vi "String-Cluster.vi"() -> ()   [LabVIEW 2012]
panel:
  out "Output":i32[](array[numeric])
  out "Input":i64[](array[numeric])
  out "Correlator Initial Data 2":T1={"[0]"=1, "Channel1 Threshold Voltage (mV)"=1, "Channel1 Pulse Front"="", "Channel2 Threshold Voltage (mV)"=1, "Channel2 Pulse Front"="", "Channel3 Threshold Voltage (mV)"=1, "Channel3 Pulse Front "="", "Channel4 Threshold Voltage (mV)"=1, "Channel4 Pulse Front "="", "Single Count Enable"={"Channel1"=FALSE, "Channel2"=FALSE, "Channel3"=FALSE, "Channel4"=FALSE}, "Single Count Max"=1, "Sum Count Enable"={"Channel1"=FALSE, "Channel2"=FALSE, "Channel3"=FALSE, "Channel4"=FALSE}, "Sum Count Max"=1, "Start-Stop1 Multyplex"={"Start Channel"="", "Stop Channel"=""}, "Stop Delay 1 (ns)"=1, "Window Length 1 (ns)"=4, "Window Offset 1 (ns) "=4, "Conditional Correlation 1"="", "Histogram Bin 1"="", "Histogram Start 1 (ns) "=4, "Start-Stop2 Multyplex "={"Start Channel"="", "Stop Channel"=""}, "Stop Delay 2 (ns)"=1, "Window Length 2 (ns) "=4, "Window Offset 2 (ns) "=4, "Conditional Correlation 2"="", "Histogram Bin 2"="", "Histogram Start 2 (ns)  "=4, "Start-Stop3 Multyplex"={"Start Channel"="", "Stop Channel"=""}, "Stop Delay 3 (ns)"=1, "Window Length 3 (ns) "=4, "Window Offset 3 (ns) "=4, "Conditional Correlation 3"="", "Histogram Bin 3"="", "Histogram Start 3 (ns) "=4, "Start-Stop4 Multyplex"={"Start Channel"="", "Stop Channel"=""}, "Stop Delay 4 (ns)"=1, "Window Length 4 (ns)  "=4, "Window Offset 4 (ns) "=4, "Conditional Correlation 4"="", "Histogram Bin 4"="", "Histogram Start 4 (ns)  "=4, "Coincidence Count Enable"={"Start-Stop1"=FALSE, "Start-Stop2"=FALSE, "Start-Stop3"=FALSE, "Start-Stop4"=FALSE}, "Coincidence Count Max"=1, "Coincidence Sum Enable 2"={"Start-Stop1"=FALSE, "Start-Stop2"=FALSE, "Start-Stop3"=FALSE, "Start-Stop4"=FALSE}, "Coincidence Sum Max"=1, "Output Channel Enable"={"Channel1"=FALSE, "Channel2"=FALSE, "Channel3"=FALSE, "Channel4"=FALSE}, "Output Channel Inversion"={"Channel1"=FALSE, "Channel2"=FALSE, "Channel3"=FALSE, "Channel4"=FALSE, "Output"=FALSE}} {"Coincidence Sum Max" min=1 max=16777215 step=1 format="%.7e"; "Coincidence Count Max" min=1 max=16777215 step=1 format="%.7e"; "Histogram Start 4 (ns)" min=0 max=120000 step=2; "Window Offset 4 (ns)" min=0 max=120000 step=2; "Window Length 4 (ns)" min=4 max=60000 step=4; "Stop Delay 4 (ns)" min=0 max=1008 step=16; "Histogram Start 3 (ns)" min=0 max=120000 step=2; "Window Offset 3 (ns)" min=0 max=120000 step=2; "Window Length 3 (ns)" min=4 max=60000 step=4; "Stop Delay 3 (ns)" min=0 max=1008 step=16; "Histogram Start 2 (ns)" min=0 max=120000 step=2; "Window Offset 2 (ns)" min=0 max=120000 step=2; "Window Length 2 (ns)" min=4 max=60000 step=4; "Stop Delay 2 (ns)" min=0 max=1008 step=16; "Histogram Start 1 (ns)" min=0 max=120000 step=2; "Window Offset 1 (ns)" min=0 max=120000 step=2; "Window Length 1 (ns)" min=4 max=60000 step=4; "Stop Delay 1 (ns)" min=0 max=1008 step=16; "Sum Count Max" min=1 max=16777215 step=1 format="%.7e"; "Single Count Max" min=1 max=16777215 step=1 format="%.7e"; "Channel4 Threshold Voltage (mV)" min=0 max=5000 step=10; "Channel3 Threshold Voltage (mV)" min=0 max=5000 step=10; "Channel2 Threshold Voltage (mV)" min=0 max=5000 step=10; "Channel1 Threshold Voltage (mV)" min=0 max=5000 step=10; "Max Exposition Time (ms)" min=1 step=1 format="%.9e"}
  out "string":string
  in  "Correlator Initial Data":T2={"Max Exposition Time (ms)"=1, "Channel1 Threshold Voltage (mV)"=1, "Channel1 Pulse Front"="", "Channel2 Threshold Voltage (mV)"=1, "Channel2 Pulse Front"="", "Channel3 Threshold Voltage (mV)"=1, "Channel3 Pulse Front "="", "Channel4 Threshold Voltage (mV)"=1, "Channel4 Pulse Front "="", "Single Count Enable"={"Channel1"=FALSE, "Channel2"=FALSE, "Channel3"=FALSE, "Channel4"=FALSE}, "Single Count Max"=1, "Sum Count Enable"={"Channel1"=FALSE, "Channel2"=FALSE, "Channel3"=FALSE, "Channel4"=FALSE}, "Sum Count Max"=1, "Start-Stop1 Multyplex"={"Start Channel"="", "Stop Channel"=""}, "Stop Delay 1 (ns)"=1, "Window Length 1 (ns)"=4, "Window Offset 1 (ns) "=4, "Conditional Correlation 1"="", "Histogram Bin 1"="", "Histogram Start 1 (ns) "=4, "Start-Stop2 Multyplex "={"Start Channel"="", "Stop Channel"=""}, "Stop Delay 2 (ns)"=1, "Window Length 2 (ns) "=4, "Window Offset 2 (ns) "=4, "Conditional Correlation 2"="", "Histogram Bin 2"="", "Histogram Start 2 (ns)  "=4, "Start-Stop3 Multyplex"={"Start Channel"="", "Stop Channel"=""}, "Stop Delay 3 (ns)"=1, "Window Length 3 (ns) "=4, "Window Offset 3 (ns) "=4, "Conditional Correlation 3"="", "Histogram Bin 3"="", "Histogram Start 3 (ns) "=4, "Start-Stop4 Multyplex"={"Start Channel"="", "Stop Channel"=""}, "Stop Delay 4 (ns)"=1, "Window Length 4 (ns)  "=4, "Window Offset 4 (ns) "=4, "Conditional Correlation 4"="", "Histogram Bin 4"="", "Histogram Start 4 (ns)  "=4, "Coincidence Count Enable"={"Start-Stop1"=FALSE, "Start-Stop2"=FALSE, "Start-Stop3"=FALSE, "Start-Stop4"=FALSE}, "Coincidence Count Max"=1, "Coincidence Sum Enable 2"={"Start-Stop1"=FALSE, "Start-Stop2"=FALSE, "Start-Stop3"=FALSE, "Start-Stop4"=FALSE}, "Coincidence Sum Max"=1, "Output Channel Enable"={"Channel1"=FALSE, "Channel2"=FALSE, "Channel3"=FALSE, "Channel4"=FALSE}, "Output Channel Inversion"={"Channel1"=FALSE, "Channel2"=FALSE, "Channel3"=FALSE, "Channel4"=FALSE, "Output"=FALSE}} {"Coincidence Sum Max" min=1 max=16777215 step=1 format="%.7e"; "Coincidence Count Max" min=1 max=16777215 step=1 format="%.7e"; "Histogram Start 4 (ns)" min=0 max=120000 step=2; "Window Offset 4 (ns)" min=0 max=120000 step=2; "Window Length 4 (ns)" min=4 max=60000 step=4; "Stop Delay 4 (ns)" min=0 max=1008 step=16; "Histogram Start 3 (ns)" min=0 max=120000 step=2; "Window Offset 3 (ns)" min=0 max=120000 step=2; "Window Length 3 (ns)" min=4 max=60000 step=4; "Stop Delay 3 (ns)" min=0 max=1008 step=16; "Histogram Start 2 (ns)" min=0 max=120000 step=2; "Window Offset 2 (ns)" min=0 max=120000 step=2; "Window Length 2 (ns)" min=4 max=60000 step=4; "Stop Delay 2 (ns)" min=0 max=1008 step=16; "Histogram Start 1 (ns)" min=0 max=120000 step=2; "Window Offset 1 (ns)" min=0 max=120000 step=2; "Window Length 1 (ns)" min=4 max=60000 step=4; "Stop Delay 1 (ns)" min=0 max=1008 step=16; "Sum Count Max" min=1 max=16777215 step=1 format="%.7e"; "Single Count Max" min=1 max=16777215 step=1 format="%.7e"; "Channel4 Threshold Voltage (mV)" min=0 max=5000 step=10; "Channel3 Threshold Voltage (mV)" min=0 max=5000 step=10; "Channel2 Threshold Voltage (mV)" min=0 max=5000 step=10; "Channel1 Threshold Voltage (mV)" min=0 max=5000 step=10; "Max Exposition Time (ms)" min=1 max=3600000000 step=1 format="%.9e"}
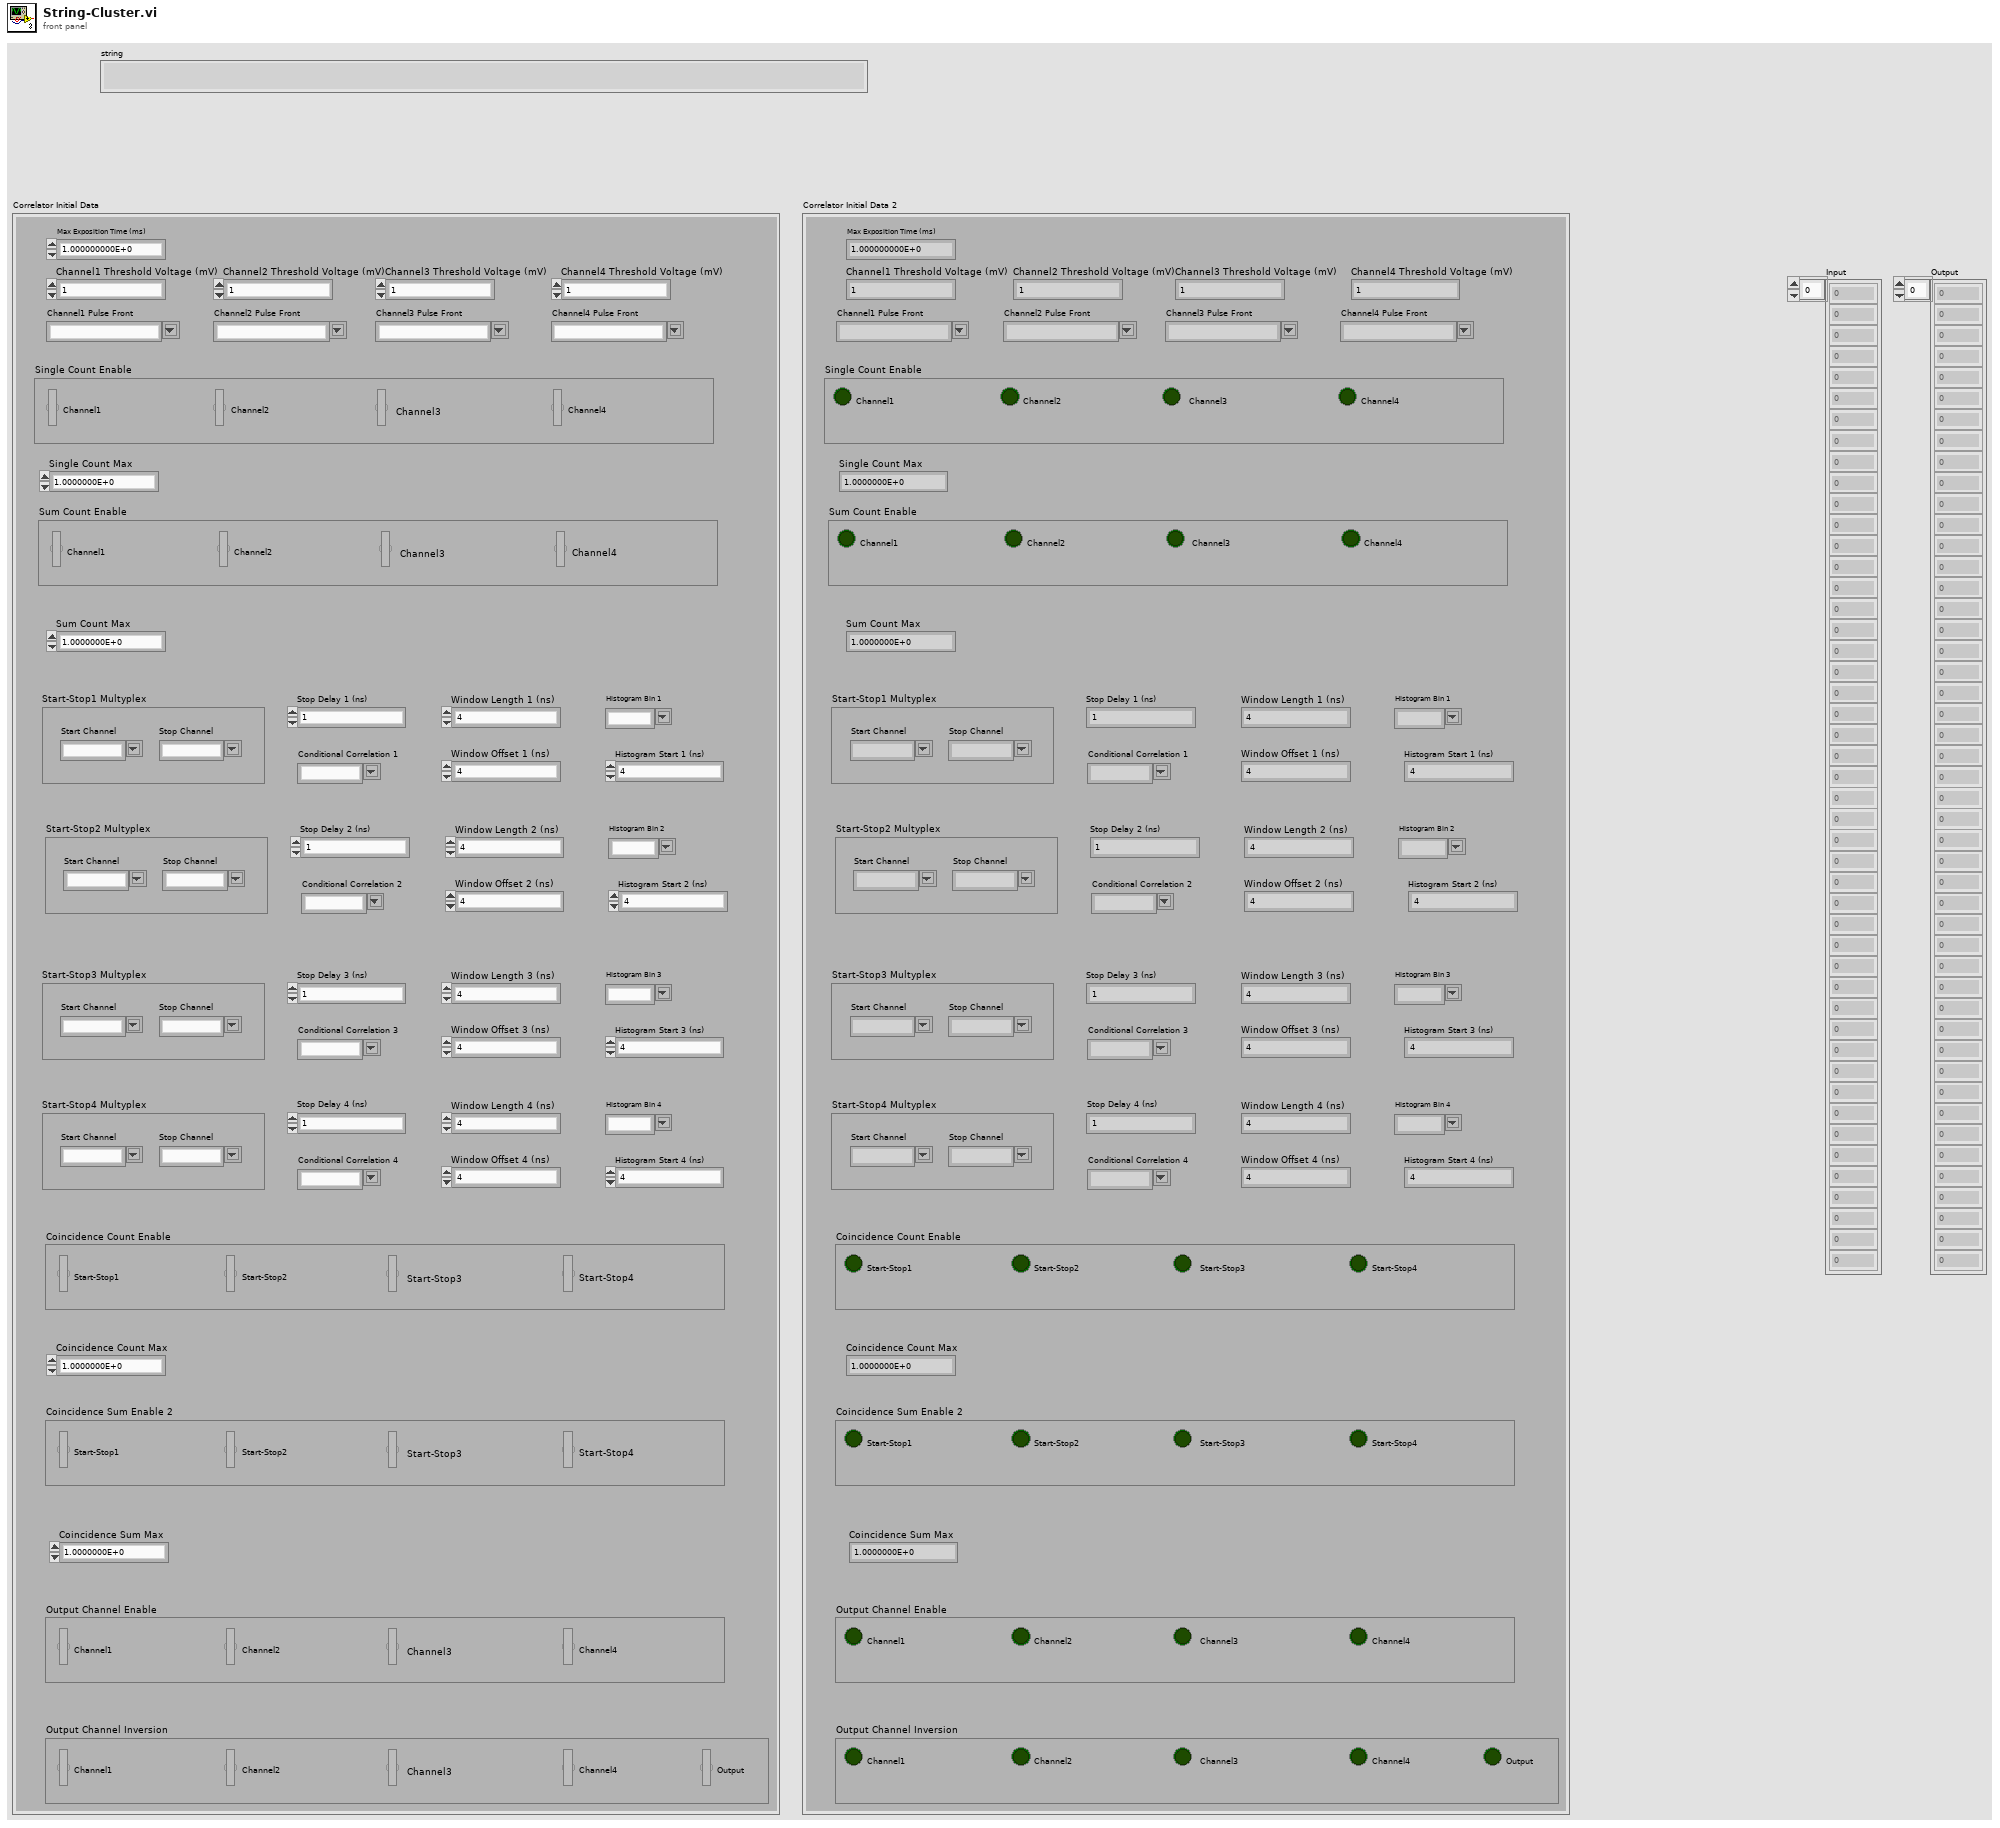
[diagram p1: front panel]
types:
  T1 = cluster{"[0]":i64, "Channel1 Threshold Voltage (mV)":i32, "Channel1 Pulse Front":string, "Channel2 Threshold Voltage (mV)":i32, "Channel2 Pulse Front":string, "Channel3 Threshold Voltage (mV)":i32, "Channel3 Pulse Front ":string, "Channel4 Threshold Voltage (mV)":i32, "Channel4 Pulse Front ":string, "Single Count Enable":cluster{"Channel1":bool, "Channel2":bool, "Channel3":bool, "Channel4":bool}, "Single Count Max":i32, "Sum Count Enable":cluster{"Channel1":bool, "Channel2":bool, "Channel3":bool, "Channel4":bool}, "Sum Count Max":i32, "Start-Stop1 Multyplex":cluster{"Start Channel":string, "Stop Channel":string}, "Stop Delay 1 (ns)":i16, "Window Length 1 (ns)":i32, "Window Offset 1 (ns) ":i32, "Conditional Correlation 1":string, "Histogram Bin 1":string, "Histogram Start 1 (ns) ":i32, "Start-Stop2 Multyplex ":cluster{"Start Channel":string, "Stop Channel":string}, "Stop Delay 2 (ns)":i16, "Window Length 2 (ns) ":i32, "Window Offset 2 (ns) ":i32, "Conditional Correlation 2":string, "Histogram Bin 2":string, "Histogram Start 2 (ns)  ":i32, "Start-Stop3 Multyplex":cluster{"Start Channel":string, "Stop Channel":string}, "Stop Delay 3 (ns)":i16, "Window Length 3 (ns) ":i32, "Window Offset 3 (ns) ":i32, "Conditional Correlation 3":string, "Histogram Bin 3":string, "Histogram Start 3 (ns) ":i32, "Start-Stop4 Multyplex":cluster{"Start Channel":string, "Stop Channel":string}, "Stop Delay 4 (ns)":i16, "Window Length 4 (ns)  ":i32, "Window Offset 4 (ns) ":i32, "Conditional Correlation 4":string, "Histogram Bin 4":string, "Histogram Start 4 (ns)  ":i32, "Coincidence Count Enable":cluster{"Start-Stop1":bool, "Start-Stop2":bool, "Start-Stop3":bool, "Start-Stop4":bool}, "Coincidence Count Max":i32, "Coincidence Sum Enable 2":cluster{"Start-Stop1":bool, "Start-Stop2":bool, "Start-Stop3":bool, "Start-Stop4":bool}, "Coincidence Sum Max":i32, "Output Channel Enable":cluster{"Channel1":bool, "Channel2":bool, "Channel3":bool, "Channel4":bool}, "Output Channel Inversion":cluster{"Channel1":bool, "Channel2":bool, "Channel3":bool, "Channel4":bool, "Output":bool}}
  T2 = cluster{"Max Exposition Time (ms)":i64, "Channel1 Threshold Voltage (mV)":i32, "Channel1 Pulse Front":string, "Channel2 Threshold Voltage (mV)":i32, "Channel2 Pulse Front":string, "Channel3 Threshold Voltage (mV)":i32, "Channel3 Pulse Front ":string, "Channel4 Threshold Voltage (mV)":i32, "Channel4 Pulse Front ":string, "Single Count Enable":cluster{"Channel1":bool, "Channel2":bool, "Channel3":bool, "Channel4":bool}, "Single Count Max":i32, "Sum Count Enable":cluster{"Channel1":bool, "Channel2":bool, "Channel3":bool, "Channel4":bool}, "Sum Count Max":i32, "Start-Stop1 Multyplex":cluster{"Start Channel":string, "Stop Channel":string}, "Stop Delay 1 (ns)":i16, "Window Length 1 (ns)":i32, "Window Offset 1 (ns) ":i32, "Conditional Correlation 1":string, "Histogram Bin 1":string, "Histogram Start 1 (ns) ":i32, "Start-Stop2 Multyplex ":cluster{"Start Channel":string, "Stop Channel":string}, "Stop Delay 2 (ns)":i16, "Window Length 2 (ns) ":i32, "Window Offset 2 (ns) ":i32, "Conditional Correlation 2":string, "Histogram Bin 2":string, "Histogram Start 2 (ns)  ":i32, "Start-Stop3 Multyplex":cluster{"Start Channel":string, "Stop Channel":string}, "Stop Delay 3 (ns)":i16, "Window Length 3 (ns) ":i32, "Window Offset 3 (ns) ":i32, "Conditional Correlation 3":string, "Histogram Bin 3":string, "Histogram Start 3 (ns) ":i32, "Start-Stop4 Multyplex":cluster{"Start Channel":string, "Stop Channel":string}, "Stop Delay 4 (ns)":i16, "Window Length 4 (ns)  ":i32, "Window Offset 4 (ns) ":i32, "Conditional Correlation 4":string, "Histogram Bin 4":string, "Histogram Start 4 (ns)  ":i32, "Coincidence Count Enable":cluster{"Start-Stop1":bool, "Start-Stop2":bool, "Start-Stop3":bool, "Start-Stop4":bool}, "Coincidence Count Max":i32, "Coincidence Sum Enable 2":cluster{"Start-Stop1":bool, "Start-Stop2":bool, "Start-Stop3":bool, "Start-Stop4":bool}, "Coincidence Sum Max":i32, "Output Channel Enable":cluster{"Channel1":bool, "Channel2":bool, "Channel3":bool, "Channel4":bool}, "Output Channel Inversion":cluster{"Channel1":bool, "Channel2":bool, "Channel3":bool, "Channel4":bool, "Output":bool}}
  T3 = cluster{"Channel1":bool, "Channel2":bool, "Channel3":bool, "Channel4":bool}
  T4 = cluster{"Start Channel":string, "Stop Channel":string}
  T5 = cluster{"Start-Stop1":bool, "Start-Stop2":bool, "Start-Stop3":bool, "Start-Stop4":bool}
  T6 = cluster{"Channel1":bool, "Channel2":bool, "Channel3":bool, "Channel4":bool, "Output":bool}
  T7 = cluster{"Channel1 Pulse Front":string, "Channel2 Pulse Front":string, "Channel3 Pulse Front ":string, "Channel4 Pulse Front ":string, "Conditional Correlation 1":string, "Histogram Bin 1":string, "Conditional Correlation 2":string, "Histogram Bin 2":string, "Conditional Correlation 3":string, "Histogram Bin 3":string, "Conditional Correlation 4":string, "Histogram Bin 4":string}
  T8 = cluster{"Channel1 Pulse Front":u32, "Channel2 Pulse Front":u32, "Channel3 Pulse Front ":u32, "Channel4 Pulse Front ":u32, "Conditional Correlation 1":u32, "Histogram Bin 1":u32, "Conditional Correlation 2":u32, "Histogram Bin 2":u32, "Conditional Correlation 3":u32, "Histogram Bin 3":u32, "Conditional Correlation 4":u32, "Histogram Bin 4":u32}
  T9 = cluster{"[0]":i64, "[1]":i64, "[2]":i64, "[3]":i64, "[4]":i64, "[5]":i64, "[6]":i64, "[7]":i64, "[8]":i64, "[9]":i64, "[10]":i64, "[11]":i64, "[12]":i64, "[13]":i64, "[14]":i64, "[15]":i64, "[16]":i64, "[17]":i64, "[18]":i64, "[19]":i64, "[20]":i64, "[21]":i64, "[22]":i64, "[23]":i64, "[24]":i64, "[25]":i64, "[26]":i64, "[27]":i64, "[28]":i64, "[29]":i64, "[30]":i64, "[31]":i64, "[32]":i64, "[33]":i64, "[34]":i64, "[35]":i64, "[36]":i64, "[37]":i64, "[38]":i64, "[39]":i64, "[40]":i64, "[41]":i64, "[42]":i64, "[43]":i64, "[44]":i64, "[45]":i64, "[46]":i64}
  T10 = cluster{"[2]":i64, "[4]":i64, "[6]":i64, "[8]":i64, "[17]":i64, "[18]":i64, "[24]":i64, "[25]":i64, "[31]":i64, "[32]":i64, "[38]":i64, "[39]":i64}
  T11 = cluster{"Boolean array[0]":bool, "Boolean array[1]":bool, "Boolean array[2]":bool, "Boolean array[3]":bool, "Boolean array[4]":bool, "Boolean array[5]":bool, "Boolean array[6]":bool, "Boolean array[7]":bool, "Boolean array[8]":bool}
  T12 = cluster{"[2]":string, "[4]":string, "[6]":string, "[8]":string, "[17]":string, "[18]":string, "[24]":string, "[25]":string, "[31]":string, "[32]":string, "[38]":string, "[39]":string}
  T13 = cluster{"Boolean array[0]":bool, "Boolean array[1]":bool, "Boolean array[2]":bool, "Boolean array[3]":bool, "Boolean array[4]":bool}
  T14 = cluster{"[0]":i64, "64bit integer":i64, "[2]":string, "64bit integer":i64, "[4]":string, "64bit integer":i64, "[6]":string, "64bit integer":i64, "[8]":string, "Output Channel Enable 2":cluster{"Channel1":bool, "Channel2":bool, "Channel3":bool, "Channel4":bool}, "[10]":i64, "Output Channel Enable 2":cluster{"Channel1":bool, "Channel2":bool, "Channel3":bool, "Channel4":bool}, "[12]":i64, "Start-Stop1 Multyplex 2":cluster{"Start Channel":string, "Stop Channel":string}, "64bit integer":i64, "64bit integer":i64, "64bit integer":i64, "[17]":string, "[18]":string, "64bit integer":i64, "Start-Stop1 Multyplex 2":cluster{"Start Channel":string, "Stop Channel":string}, "64bit integer":i64, "64bit integer":i64, "64bit integer":i64, "[24]":string, "[25]":string, "64bit integer":i64, "Start-Stop1 Multyplex 2":cluster{"Start Channel":string, "Stop Channel":string}, "64bit integer":i64, "64bit integer":i64, "64bit integer":i64, "[31]":string, "[32]":string, "64bit integer":i64, "Start-Stop1 Multyplex 2":cluster{"Start Channel":string, "Stop Channel":string}, "64bit integer":i64, "64bit integer":i64, "64bit integer":i64, "[38]":string, "[39]":string, "64bit integer":i64, "Output Channel Enable 2":cluster{"Channel1":bool, "Channel2":bool, "Channel3":bool, "Channel4":bool}, "[42]":i64, "Output Channel Enable 2":cluster{"Channel1":bool, "Channel2":bool, "Channel3":bool, "Channel4":bool}, "[44]":i64, "Output Channel Enable 2":cluster{"Channel1":bool, "Channel2":bool, "Channel3":bool, "Channel4":bool}, cluster{"Boolean array[0]":bool, "Boolean array[1]":bool, "Boolean array[2]":bool, "Boolean array[3]":bool, "Boolean array[4]":bool}}
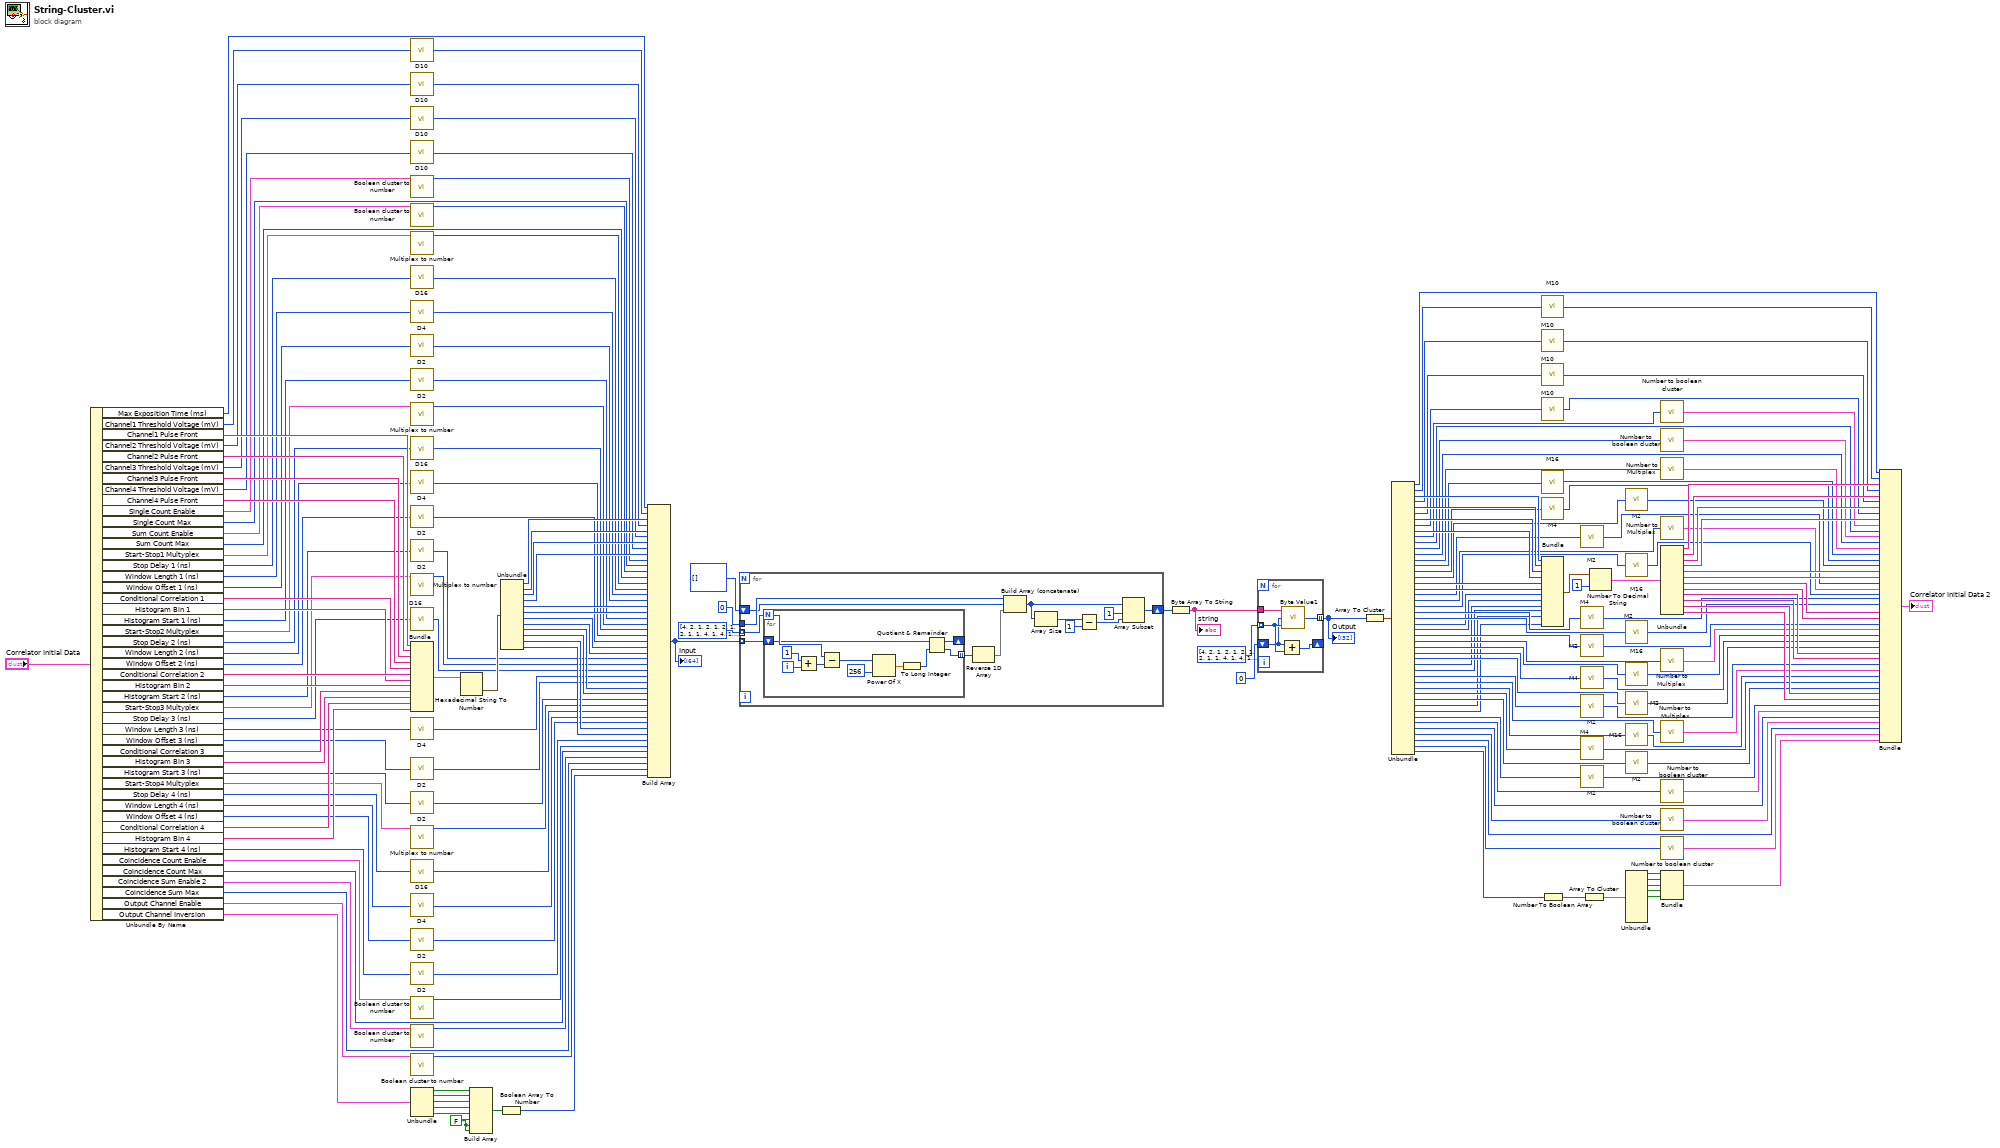
[diagram p0: block diagram]
diagram:
  w152 = FALSE ("element")
  n1 = Unbundle By Name("Correlator Initial Data") -> ("Max Exposition Time (ms)"=w180:i64, "Channel1 Threshold Voltage (mV)"=w179:i32, "Channel1 Pulse Front"=w209:string, "Channel2 Threshold Voltage (mV)"=w178:i32, "Channel2 Pulse Front"=w208:string, "Channel3 Threshold Voltage (mV)"=w177:i32, "Channel3 Pulse Front"=w207:string, "Channel4 Threshold Voltage (mV)"=w176:i32, "Channel4 Pulse Front"=w206:string, "Single Count Enable"=w122:T3, "Single Count Max"=w175:i32, "Sum Count Enable"=w121:T3, "Sum Count Max"=w174:i32, "Start-Stop1 Multyplex"=w185:T4, "Stop Delay 1 (ns)"=w173:i16, "Window Length 1 (ns)"=w172:i32, "Window Offset 1 (ns)"=w171:i32, "Conditional Correlation 1"=w205:string, "Histogram Bin 1"=w204:string, "Histogram Start 1 (ns)"=w170:i32, "Start-Stop2 Multyplex"=w183:T4, "Stop Delay 2 (ns)"=w169:i16, "Window Length 2 (ns)"=w168:i32, "Window Offset 2 (ns)"=w167:i32, "Conditional Correlation 2"=w203:string, "Histogram Bin 2"=w202:string, "Histogram Start 2 (ns)"=w166:i32, "Start-Stop3 Multyplex"=w181:T4, "Stop Delay 3 (ns)"=w165:i16, "Window Length 3 (ns)"=w164:i32, "Window Offset 3 (ns)"=w163:i32, "Conditional Correlation 3"=w201:string, "Histogram Bin 3"=w200:string, "Histogram Start 3 (ns)"=w162:i32, "Start-Stop4 Multyplex"=w186:T4, "Stop Delay 4 (ns)"=w161:i16, "Window Length 4 (ns)"=w160:i32, "Window Offset 4 (ns)"=w159:i32, "Conditional Correlation 4"=w199:string, "Histogram Bin 4"=w198:string, "Histogram Start 4 (ns)"=w158:i32, "Coincidence Count Enable"=w125:T5, "Coincidence Count Max"=w70:i32, "Coincidence Sum Enable 2"=w123:T5, "Coincidence Sum Max"=w72:i32, "Output Channel Enable"=w124:T3, "Output Channel Inversion"=w151:T6)
  n2 = call "D10.vi"("x"=w179) -> ("64bit integer"=w104:i64)
  n3 = call "D10.vi"("x"=w178) -> ("64bit integer"=w103:i64)
  n4 = call "D10.vi"("x"=w177) -> ("64bit integer"=w102:i64)
  n5 = call "D10.vi"("x"=w176) -> ("64bit integer"=w101:i64)
  n6 = call "Boolean cluster to number.vi"("Output Channel Enable"=w122) -> ("Numeric"=w188:u32)  [unwired: 10 in]
  n7 = call "Boolean cluster to number.vi"("Output Channel Enable"=w121) -> ("Numeric"=w187:u32)  [unwired: 10 in]
  n8 = call "Multiplex to number.vi"("Start-Stop4 Multyplex"=w185) -> ("Numeric"=w184:u32)  [unwired: 10 in]
  n9 = call "D16.vi"("x"=w173) -> ("64bit integer"=w100:i64)
  n10 = call "D4.vi"("x"=w172) -> ("64bit integer"=w99:i64)
  n11 = call "D2.vi"("x"=w171) -> ("64bit integer"=w98:i64)
  n12 = call "D2.vi"("x"=w170) -> ("64bit integer"=w97:i64)
  n13 = call "Multiplex to number.vi"("Start-Stop4 Multyplex"=w183) -> ("Numeric"=w182:u32)  [unwired: 10 in]
  n14 = call "D16.vi"("x"=w169) -> ("64bit integer"=w96:i64)
  n15 = call "D4.vi"("x"=w168) -> ("64bit integer"=w95:i64)
  n16 = call "D2.vi"("x"=w167) -> ("64bit integer"=w94:i64)
  n17 = call "D2.vi"("x"=w166) -> ("64bit integer"=w54:i64)
  n18 = call "Multiplex to number.vi"("Start-Stop4 Multyplex"=w181) -> ("Numeric"=w55:u32)  [unwired: 10 in]
  n19 = call "D16.vi"("x"=w165) -> ("64bit integer"=w56:i64)
  n20 = Bundle("Channel1 Pulse Front"=w209, "Channel2 Pulse Front"=w208, "Channel3 Pulse Front"=w207, "Channel4 Pulse Front"=w206, "Conditional Correlation 1"=w205, "Histogram Bin 1"=w204, "Conditional Correlation 2"=w203, "Histogram Bin 2"=w202, "Conditional Correlation 3"=w201, "Histogram Bin 3"=w200, "Conditional Correlation 4"=w199, "Histogram Bin 4"=w198) -> (w197:T7)  [unwired: 1 in]
  n21 = call "D4.vi"("x"=w164) -> ("64bit integer"=w57:i64)
  n22 = call "D2.vi"("x"=w163) -> ("64bit integer"=w58:i64)
  n23 = call "D2.vi"("x"=w162) -> ("64bit integer"=w61:i64)
  n24 = call "Multiplex to number.vi"("Start-Stop4 Multyplex"=w186) -> ("Numeric"=w62:u32)  [unwired: 10 in]
  n25 = call "D16.vi"("x"=w161) -> ("64bit integer"=w63:i64)
  n26 = call "D4.vi"("x"=w160) -> ("64bit integer"=w64:i64)
  n27 = call "D2.vi"("x"=w159) -> ("64bit integer"=w65:i64)
  n28 = call "D2.vi"("x"=w158) -> ("64bit integer"=w68:i64)
  n29 = call "Boolean cluster to number.vi"("Output Channel Enable"=w125) -> ("Numeric"=w69:u32)  [unwired: 10 in]
  n30 = call "Boolean cluster to number.vi"("Output Channel Enable"=w123) -> ("Numeric"=w71:u32)  [unwired: 10 in]
  n31 = call "Boolean cluster to number.vi"("Output Channel Enable"=w124) -> ("Numeric"=w73:u32)  [unwired: 10 in]
  n32 = Unbundle(w151) -> ("Channel1"=w154:bool, "Channel2"=w155:bool, "Channel3"=w156:bool, "Channel4"=w157:bool, "Output"=w150:bool)
  n33 = Hexadecimal String To Number(string=w197) -> (number=w196:T8)  [unwired: 2 in, 1 out]
  n34 = Build Array(w154, w155, w156, w157, w150, w152, w152, w152) -> (w153:bool[])
  n35 = Boolean Array To Number(Boolean array=w153) -> (number=w74:u32)
  n36 = Unbundle(w196) -> ("Channel1 Pulse Front"=w194:u32, "Channel2 Pulse Front"=w193:u32, "Channel3 Pulse Front"=w192:u32, "Channel4 Pulse Front"=w191:u32, "Conditional Correlation 1"=w190:u32, "Histogram Bin 1"=w189:u32, "Conditional Correlation 2"=w52:u32, "Histogram Bin 2"=w53:u32, "Conditional Correlation 3"=w59:u32, "Histogram Bin 3"=w60:u32, "Conditional Correlation 4"=w66:u32, "Histogram Bin 4"=w67:u32)
  n37 = Build Array(w180, w104, w194, w103, w193, w102, w192, w101, w191, w188, w175, w187, w174, w184, w100, w99, w98, w190, w189, w97, w182, w96, w95, w94, w52, w53, w54, w55, w56, w57, w58, w59, w60, w61, w62, w63, w64, w65, w66, w67, w68, w69, w70, w71, w72, w73, w74) -> (w51:i64[])
  "Input" <- w51
  n38 = for {
    tunnel: i8[] [4, 2, 1, 2, 1, 2, 1, 2, 1, 1, 4, 1, 4, 1, 1, 2, 2, 1, 1, 2, 1, 1, 2, 2, 1, 1, 2, 1, 1, 2, 2, 1, 1, 2, 1, 1, 2, 2, 1, 1, 2, 1, 4, 1, 4, 1, 1] ("Length array") -> [w221] mode=indexing
    tunnel: w51 -> [w220] mode=indexing
    shift-right: [w213] -> w107
    shift-left: i8[] [] -> [w218]
    tunnel: 0 -> [w219]
    n39 = for {
      N: w221 -> [w232]
      tunnel: [w222] -> w211 mode=indexing
      shift-right: [w225] -> _
      shift-left: w220 -> [w226]
      i -> [w231]
      n40 = Add(x=1, y=w231) -> (x+y=w229:i32)
      n41 = Subtract(x=w232, y=w229) -> (x-y=w228:i32)
      n42 = Power Of X(1:256 ("x"), 2:w228) -> (0:w224:dbl)
      n43 = To Long Integer(number=w224) -> (32bit integer=w223:i32)
      n44 = Quotient & Remainder(x=w226, y=w223) -> (x-y*floor(x/y)=w225:i64, floor(x/y)=w222:i64)
    }
    n45 = Reverse 1D Array(array=w211) -> (reversed array=w210:i64[])
    n46 = Build Array (concatenate)(w219, w218, w210) -> (w212:i64[])
    n47 = Array Size(array=w212) -> (size(s)=w216:i32)
    n48 = Subtract(x=w216, y=1) -> (x-y=w214:i32)
    n49 = Array Subset(array=w212, index=1, length=w214) -> (w213:i64[])
  }
  n50 = Byte Array To String(unsigned byte array=w107) -> (string=w106:string)
  "string" <- w106
  n51 = for {
    tunnel: i8[] [4, 2, 1, 2, 1, 2, 1, 2, 1, 1, 4, 1, 4, 1, 1, 2, 2, 1, 1, 2, 1, 1, 2, 2, 1, 1, 2, 1, 1, 2, 2, 1, 1, 2, 1, 1, 2, 2, 1, 1, 2, 1, 4, 1, 4, 1, 1] ("Length array") -> [w236] mode=indexing
    tunnel: w106 -> [w237]
    shift-right: [w235] -> _
    shift-left: i8 0 -> [w234]
    tunnel: [w233] -> w50 mode=indexing
    n52 = Add(x=w234, y=w236) -> (x+y=w235:i8)
    n53 = call "Byte Value1.vi"("Length"=w236, "Offset"=w234, "string"=w237) -> ("Value"=w233:i64)
  }
  "Output" <- w50
  n54 = Array To Cluster(array=w50) -> (cluster=w49:T9)
  n55 = Unbundle(w49) -> ("[0]"=w48:i64, "[1]"=w47:i64, "[2]"=w46:i64, "[3]"=w45:i64, "[4]"=w44:i64, "[5]"=w43:i64, "[6]"=w42:i64, "[7]"=w41:i64, "[8]"=w40:i64, "[9]"=w39:i64, "[10]"=w38:i64, "[11]"=w37:i64, "[12]"=w36:i64, "[13]"=w35:i64, "[14]"=w34:i64, "[15]"=w33:i64, "[16]"=w32:i64, "[17]"=w31:i64, "[18]"=w30:i64, "[19]"=w29:i64, "[20]"=w28:i64, "[21]"=w27:i64, "[22]"=w26:i64, "[23]"=w25:i64, "[24]"=w24:i64, "[25]"=w23:i64, "[26]"=w22:i64, "[27]"=w21:i64, "[28]"=w20:i64, "[29]"=w19:i64, "[30]"=w18:i64, "[31]"=w17:i64, "[32]"=w16:i64, "[33]"=w15:i64, "[34]"=w14:i64, "[35]"=w12:i64, "[36]"=w11:i64, "[37]"=w10:i64, "[38]"=w9:i64, "[39]"=w8:i64, "[40]"=w7:i64, "[41]"=w6:i64, "[42]"=w5:i64, "[43]"=w4:i64, "[44]"=w3:i64, "[45]"=w2:i64, "[46]"=w1:i64)
  n56 = call "M10.vi"("x"=w47) -> ("64bit integer"=w93:i64)
  n57 = call "M10.vi"("x"=w45) -> ("64bit integer"=w92:i64)
  n58 = call "M10.vi"("x"=w43) -> ("64bit integer"=w91:i64)
  n59 = call "M10.vi"("x"=w41) -> ("64bit integer"=w90:i64)
  n60 = call "M16.vi"("x"=w34) -> ("64bit integer"=w89:i64)
  n61 = call "M4.vi"("x"=w33) -> ("64bit integer"=w88:i64)
  n62 = Bundle("[2]"=w46, "[4]"=w44, "[6]"=w42, "[8]"=w40, "[17]"=w31, "[18]"=w30, "[24]"=w24, "[25]"=w23, "[31]"=w17, "[32]"=w16, "[38]"=w9, "[39]"=w8) -> (w147:T10)  [unwired: 1 in]
  n63 = Number To Boolean Array(number=w1) -> (Boolean array=w133:bool[])
  n64 = call "M2.vi"("x"=w29) -> ("64bit integer"=w86:i64)
  n65 = call "M4.vi"("x"=w26) -> ("64bit integer"=w84:i64)
  n66 = call "M2.vi"("x"=w22) -> ("64bit integer"=w82:i64)
  n67 = call "M4.vi"("x"=w19) -> ("64bit integer"=w80:i64)
  n68 = call "M2.vi"("x"=w15) -> ("64bit integer"=w78:i64)
  n69 = call "M4.vi"("x"=w11) -> ("64bit integer"=w76:i64)
  n70 = call "M2.vi"("x"=w7) -> ("64bit integer"=w75:i64)
  n71 = Array To Cluster(array=w133) -> (cluster=w132:T11)
  n72 = Number To Decimal String(number=w147, width (-)=i16 1) -> (decimal integer string=w146:T12)
  n73 = call "M2.vi"("x"=w32) -> ("64bit integer"=w87:i64)
  n74 = call "M16.vi"("x"=w27) -> ("64bit integer"=w85:i64)
  n75 = call "M2.vi"("x"=w25) -> ("64bit integer"=w83:i64)
  n76 = call "M16.vi"("x"=w20) -> ("64bit integer"=w81:i64)
  n77 = call "M2.vi"("x"=w18) -> ("64bit integer"=w79:i64)
  n78 = call "M16.vi"("x"=w12) -> ("64bit integer"=w77:i64)
  n79 = call "M2.vi"("x"=w10) -> ("64bit integer"=w13:i64)
  n80 = Unbundle(w132) -> ("Boolean array[0]"=w131:bool, "Boolean array[1]"=w130:bool, "Boolean array[2]"=w129:bool, "Boolean array[3]"=w128:bool, "Boolean array[4]"=w127:bool)  [unwired: 4 out]
  n81 = call "Number to boolean cluster.vi"("Numeric"=w39) -> ("Output Channel Enable 2"=w117:T3)
  n82 = call "Number to boolean cluster.vi"("Numeric"=w37) -> ("Output Channel Enable 2"=w116:T3)
  n83 = call "Number to Multiplex.vi"("Numeric"=w35) -> ("Start-Stop1 Multyplex 2"=w115:T4)
  n84 = call "Number to Multiplex.vi"("Numeric"=w28) -> ("Start-Stop1 Multyplex 2"=w114:T4)
  n85 = Unbundle(w146) -> ("[2]"=w145:string, "[4]"=w144:string, "[6]"=w143:string, "[8]"=w142:string, "[17]"=w141:string, "[18]"=w140:string, "[24]"=w139:string, "[25]"=w138:string, "[31]"=w137:string, "[32]"=w136:string, "[38]"=w135:string, "[39]"=w134:string)
  n86 = call "Number to Multiplex.vi"("Numeric"=w21) -> ("Start-Stop1 Multyplex 2"=w113:T4)
  n87 = call "Number to Multiplex.vi"("Numeric"=w14) -> ("Start-Stop1 Multyplex 2"=w112:T4)
  n88 = call "Number to boolean cluster.vi"("Numeric"=w6) -> ("Output Channel Enable 2"=w118:T3)
  n89 = call "Number to boolean cluster.vi"("Numeric"=w4) -> ("Output Channel Enable 2"=w119:T3)
  n90 = call "Number to boolean cluster.vi"("Numeric"=w2) -> ("Output Channel Enable 2"=w120:T3)
  n91 = Bundle("Boolean array[0]"=w131, "Boolean array[1]"=w130, "Boolean array[2]"=w129, "Boolean array[3]"=w128, "Boolean array[4]"=w127) -> (w126:T13)  [unwired: 1 in]
  n92 = Bundle("[0]"=w48, "64bit integer"=w93, "[2]"=w145, "64bit integer"=w92, "[4]"=w144, "64bit integer"=w91, "[6]"=w143, "64bit integer"=w90, "[8]"=w142, "Output Channel Enable 2"=w117, "[10]"=w38, "Output Channel Enable 2"=w116, "[12]"=w36, "Start-Stop1 Multyplex 2"=w115, "64bit integer"=w89, "64bit integer"=w88, "64bit integer"=w87, "[17]"=w141, "[18]"=w140, "64bit integer"=w86, "Start-Stop1 Multyplex 2"=w114, "64bit integer"=w85, "64bit integer"=w84, "64bit integer"=w83, "[24]"=w139, "[25]"=w138, "64bit integer"=w82, "Start-Stop1 Multyplex 2"=w113, "64bit integer"=w81, "64bit integer"=w80, "64bit integer"=w79, "[31]"=w137, "[32]"=w136, "64bit integer"=w78, "Start-Stop1 Multyplex 2"=w112, "64bit integer"=w77, "64bit integer"=w76, "64bit integer"=w13, "[38]"=w135, "[39]"=w134, "64bit integer"=w75, "Output Channel Enable 2"=w118, "[42]"=w5, "Output Channel Enable 2"=w119, "[44]"=w3, "Output Channel Enable 2"=w120, w126) -> (→"Correlator Initial Data 2":T14)  [unwired: 1 in]
